vi "Yokogawa WT300 Series Measure Integrate.vi"() -> ()   [LabVIEW 2016]
doc: "This example shows how to measure the integrate data."
uses:
  Public/Utility/Function/Create Function String (Integrate).vi
  Public/Data/Read Measurement (Normal).vi
  Yokogawa WT300 Series.lvlib
panel:
  in  "Element (1: 1)":i32(ring)=1 items=["1"=1, "2"=2, "3"=3, "Sigma A"=4]
  out "Function":string[](array[string])
  out "Measurement":dbl[](array[numeric])
  in  "Stop":bool
  in  "Update Rate (500ms)":dbl(ring)=0.5 items=["100m"=0.1, "250m"=0.25, "500m"=0.5, "1"=1.0, "2"=2.0, "5"=5.0]
  in  "Timeout (10000 ms)":i32=10000 min=1
  in  "VISA resource name":refnum<visa-resource-name>
  # "(c) 2013 Yokogawa Meters & Instruments Corporation.  All rights reserved."
  # "WT300 SERIES POWER ANALYZER"
  # "s"
  # "ms"
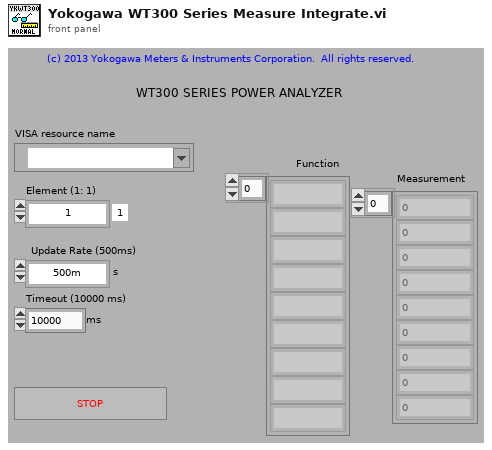
[diagram p1: front panel]
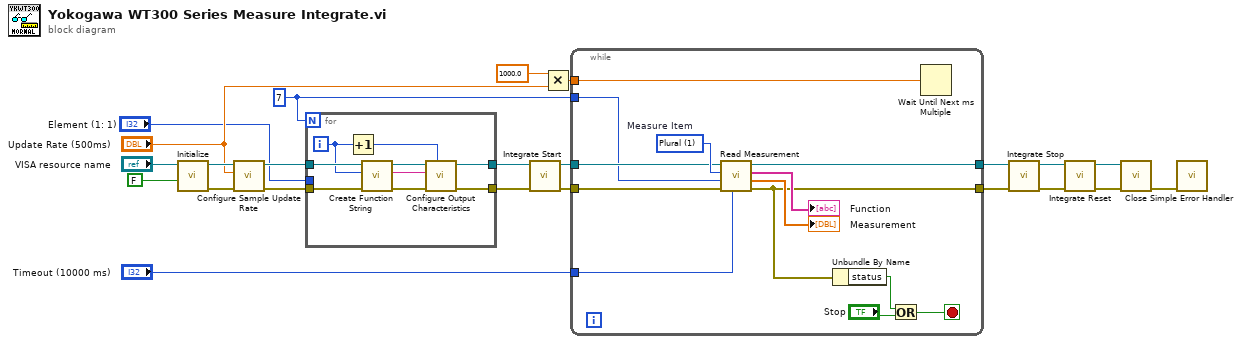
[diagram p0: block diagram]
diagram:
  w15 = 7
  n1 = call "Initialize.vi"("Reset (True)"=FALSE ("Reset? (True)"), "VISA resource name"="VISA resource name") -> ("error out"=w17:errorcluster, "VISA resource name out"=w19:refnum<visa-resource-name>)  [unwired: 7 in, 1 out]
  n2 = call "Configure Sample Update Rate.vi"("error in (no error)"=w17, "Update Rate (500m s)"="Update Rate (500ms)", "VISA resource name"=w19) -> ("error out"=w16:errorcluster, "VISA resource name out"=w18:refnum<visa-resource-name>)  [unwired: 7 in]
  n3 = for {
    N: w15 -> [_]
    tunnel: [w32] -> w3
    tunnel: [w31] -> w2
    tunnel: "Element (1: 1)" -> [_]
    tunnel: w18 -> [w27]
    tunnel: w16 -> [w26]
    i -> [w25]
    n4 = Increment(x=w25) -> (x+1=w24:i32)
    n5 = call-poly "Create Function String.vi"("error in (no error)"=w26, "Function (0: Time)"=w25, "VISA resource name"=w27) -> ("error out"=w28:errorcluster, "Function String"=w30:string, "VISA resource name out"=w29:refnum<visa-resource-name>)  [unwired: 6 in]
    n6 = call "Configure Output Characteristics.vi"("Item (1)"=w24, "error in (no error)"=w28, "Function (Empty)"=w30, "VISA resource name"=w29) -> ("error out"=w31:errorcluster, "VISA resource name out"=w32:refnum<visa-resource-name>)  [unwired: 6 in]
  }
  n7 = call "Integrate Start.vi"("error in (no error)"=w2, "VISA resource name"=w3) -> ("error out"=w13:errorcluster, "VISA resource name out"=w14:refnum<visa-resource-name>)  [unwired: 8 in]
  n8 = Multiply(x=1000.0, y="Update Rate (500ms)") -> (x*y=w9:dbl)
  n9 = while {
    tunnel: [w34] -> w12
    tunnel: [w33] -> w11
    tunnel: "Timeout (10000 ms)" -> [w45]
    tunnel: w14 -> [w43]
    tunnel: w13 -> [w42]
    tunnel: w15 -> [w41]
    tunnel: w9 -> [w35]
    stop <- w38 stop-if-true
    w44 = 1 items=["One", "Plural"]  # Measure Item
    n10 = call-poly "Read Measurement.vi"("Timeout (10000 ms)"=w45, "error in (no error)"=w42, "Number of Item (15)"=w41, "Measure Item (1: Plural)"=w44, "VISA resource name"=w43) -> ("error out"=w33:errorcluster, "Measurement"=→"Measurement":dbl[], "Function"=→"Function":string[], "VISA resource name out"=w34:refnum<visa-resource-name>)  [unwired: 3 in]
    n11 = Unbundle By Name ("名前でバンドル解除")(w33) -> ("status"=w39:bool)
    n12 = Or(x=w39, y="Stop") -> (x .or. y?=w38:bool)
    n13 = Wait Until Next ms Multiple(millisecond multiple=w35) -> ()  [unwired: 1 out]
  }
  n14 = call "Integrate Stop.vi"("error in (no error)"=w11, "VISA resource name"=w12) -> ("error out"=w5:errorcluster, "VISA resource name out"=w7:refnum<visa-resource-name>)  [unwired: 8 in]
  n15 = call "Integrate Reset.vi"("error in (no error)"=w5, "VISA resource name"=w7) -> ("error out"=w4:errorcluster, "VISA resource name out"=w6:refnum<visa-resource-name>)  [unwired: 8 in]
  n16 = call "Close.vi"("error in (no error)"=w4, "VISA resource name"=w6) -> ("error out"=w23:errorcluster)  [unwired: 9 in]
  n17 = call <vilib>:"Simple Error Handler.vi"("error in (no error)"=w23) -> ()  [unwired: 4 in, 5 out]
